vi "Drive.vi"(9 "JoystickDevRef 2":T1, 10 "JoystickDevRef":T1, 11 "RobotDriveDevRef":T3={"DevStatus"={"status"=FALSE, "code"=0, "source"=""}, "Motors[]"=[], "Square Inputs"=FALSE, "Max Output"=1.0}) -> (1 "JoystickDevRef 4":T1, 2 "JoystickDevRef 3":T1, 3 "RobotDriveDevRef 2":T3={"DevStatus"={"status"=FALSE, "code"=0, "source"=""}, "Motors[]"=[], "Square Inputs"=FALSE, "Max Output"=1.0})   [LabVIEW 2019]
uses:
  <vilib>/Rock Robotics/WPI/Joystick/WPI_JoystickDevRef.ctl
  <vilib>/Rock Robotics/WPI/Joystick/WPI_JoystickDeviceEnum.ctl
  <vilib>/Rock Robotics/WPI/RobotDrive/WPI_RobotDriveDevRef.ctl
  <vilib>/Rock Robotics/WPI/MotorControl/WPI_MotorControlDeviceRef.ctl
  <vilib>/Rock Robotics/WPI/MotorControl/WPI_MotorControlType.ctl
  <vilib>/Rock Robotics/SystemInterfaces/DIO/FPGA_DIOPWMChannel.ctl
  <vilib>/Rock Robotics/WPI/PWM/WPI_PWMDeadband.ctl
  <vilib>/Rock Robotics/SystemInterfaces/DIO/FPGA_DIOChannel.ctl
  Robot Global Data.vi
  <vilib>/Rock Robotics/WPI/Utilities/WPI_GetSetVariantRefNum.vi
  <vilib>/Rock Robotics/Network Tables/NT Read Number.vi
  <vilib>/Rock Robotics/WPI/RobotDrive/WPI_RobotDriveArcadeDrive_Standard(NoSaturation).vi
panel:
  in  "Double":dbl=0.5
  in  "Plus":dbl=0.2
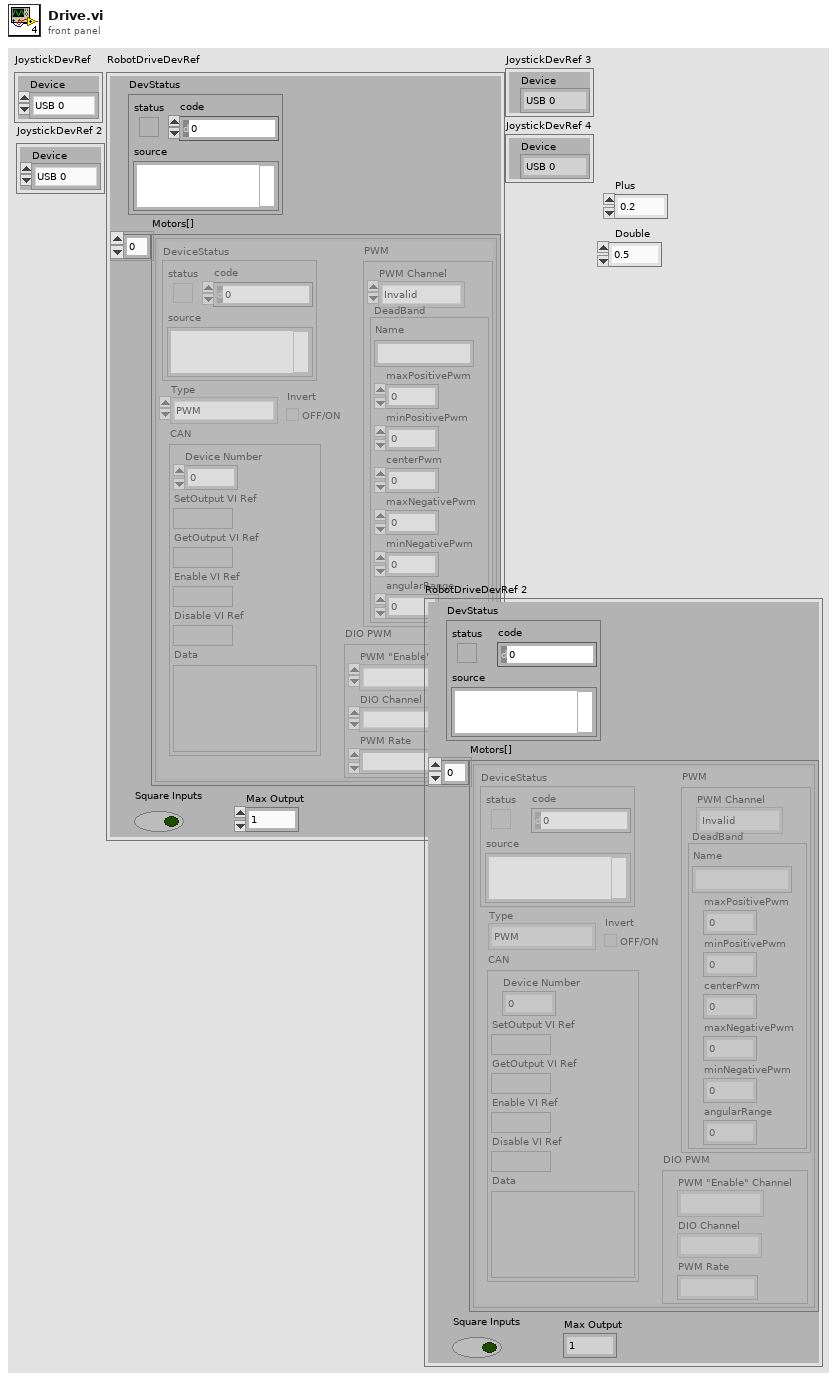
[diagram p1: front panel]
types:
  T1 = typedef "WPI_JoystickDevRef.ctl" = cluster{"Device":T2}
  T2 = typedef "WPI_JoystickDeviceEnum.ctl" = enum16{"USB 0", "USB 1", "USB 2", "USB 3", "USB 4", "USB 5"}
  T3 = typedef "WPI_RobotDriveDevRef.ctl" = cluster{"DevStatus":errorcluster, "Motors[]":T4[], "Square Inputs":bool, "Max Output":dbl}
  T4 = typedef "WPI_MotorControlDeviceRef.ctl" = cluster{"DeviceStatus":errorcluster, "Type":T5, "PWM":cluster{"PWM Channel":T6, "DeadBand":T7}, "CAN":cluster{"Device Number":u8, "SetOutput VI Ref":variant, "GetOutput VI Ref":variant, "Enable VI Ref":variant, "Disable VI Ref":variant, "Data":variant}, "Invert":bool, "DIO PWM":cluster{"PWM \"Enable\" Channel":T6, "DIOChannel":T8, "PWM Rate":dbl}}
  T5 = typedef "WPI_MotorControlType.ctl" = enum16{"PWM", "CAN", "DIO PWM"}
  T6 = typedef "FPGA_DIOPWMChannel.ctl" = enum8{"PWM 0", "PWM 1", "PWM 2", "PWM 3", "PWM 4", "PWM 5", "PWM 6", "PWM 7", "PWM 8", "PWM 9", "PWM MXP 0", "PWM MXP 1", "PWM MXP 2", "PWM MXP 3", "PWM MXP 4", "PWM MXP 5", "PWM MXP 6", "PWM MXP 7", "PWM MXP 8", "PWM MXP 9", "Invalid"}
  T7 = typedef "WPI_PWMDeadband.ctl" = cluster{"Name":string, "maxPositivePwm":i32, "minPositivePwm":i32, "centerPwm":i32, "maxNegativePwm":i32, "minNegativePwm":i32, "angularRange":u16}
  T8 = typedef "FPGA_DIOChannel.ctl" = enum8{"DIO 0", "DIO 1", "DIO 2", "DIO 3", "DIO 4", "DIO 5", "DIO 6", "DIO 7", "DIO 8", "DIO 9", "DIO MXP 0", "DIO MXP 1", "DIO MXP 2", "DIO MXP 3", "DIO MXP 4", "DIO MXP 5", "DIO MXP 6", "DIO MXP 7", "DIO MXP 8", "DIO MXP 9", "DIO MXP 10", "DIO MXP 11", "DIO MXP 12", "DIO MXP 13", "DIO MXP 14", "DIO MXP 15", "SPI Port CS1", "SPI Port CS2", "SPI Port CS3", "SPI Port MISO", "SPI Port MOSI", "Invalid"}
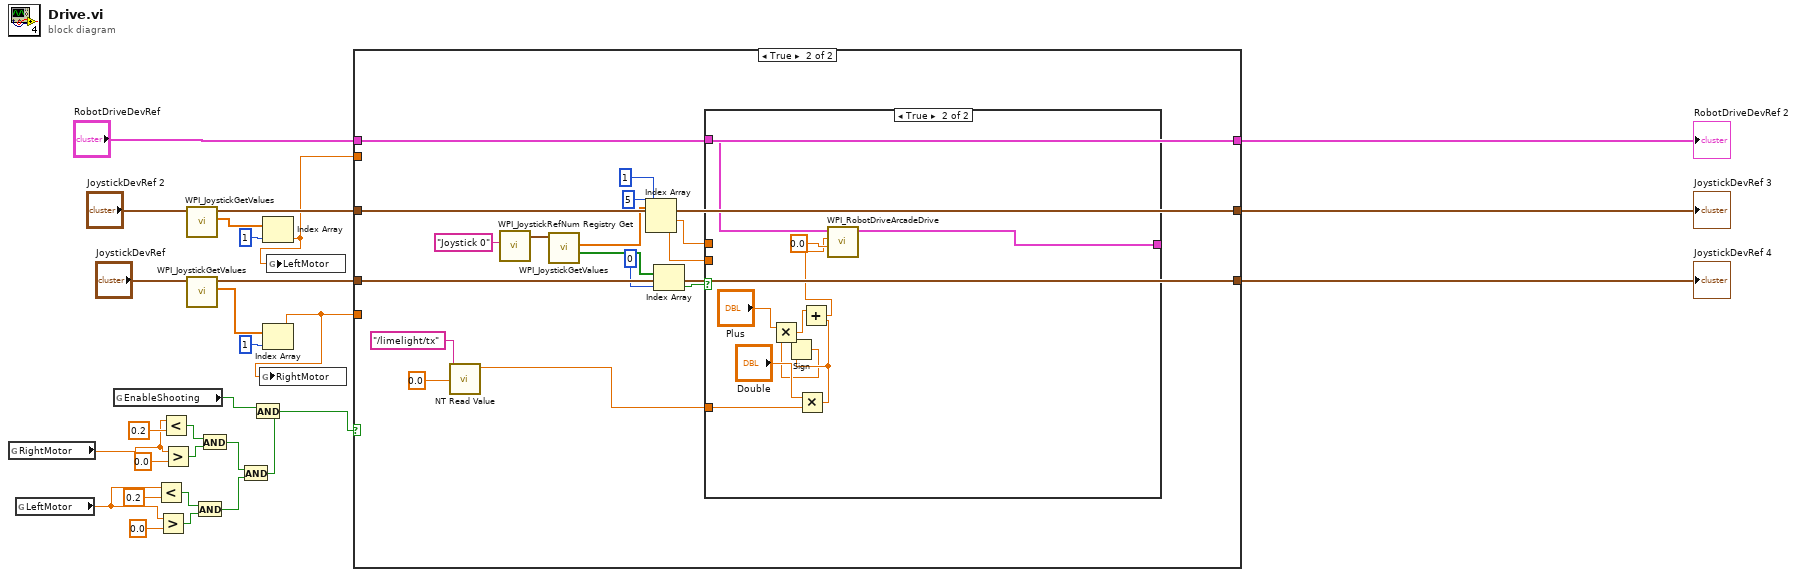
[diagram p0: block diagram]
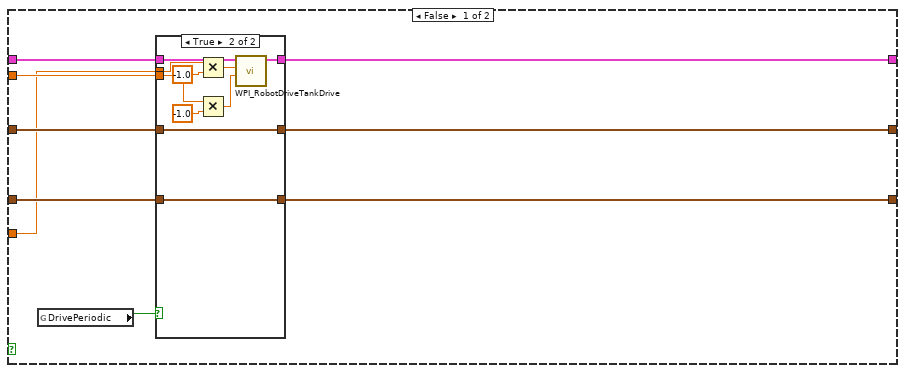
[diagram p2: hidden frame]
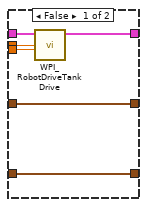
[diagram p3: hidden frame]
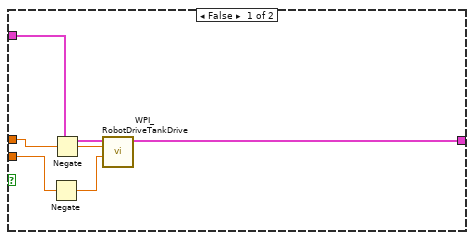
[diagram p4: hidden frame]
diagram:
  n1 = global read "Robot Global Data.vi" "RightMotor"() -> (w5:dbl)
  n2 = global read "Robot Global Data.vi" "LeftMotor"() -> (w11:dbl)
  n3 = global read "Robot Global Data.vi" "EnableShooting"() -> (w18:bool)
  n4 = Less?(x=w11, y=0.2) -> (x < y?=w12:bool)
  n5 = Greater?(x=w11, y=0.0) -> (0:w13:bool)
  n6 = Less?(x=w5, y=0.2) -> (x < y?=w7:bool)
  n7 = Greater?(x=w5, y=0.0) -> (0:w8:bool)
  n8 = call <vilib>:"WPI_JoystickGetValues.vi"("JoystickDevRef"="JoystickDevRef 2") -> ("Axes"=w28:dbl[], "JoystickDevRef"=w25:T1)  [unwired: 6 in, 3 out]
  n9 = call <vilib>:"WPI_JoystickGetValues.vi"("JoystickDevRef"="JoystickDevRef") -> ("Axes"=w29:dbl[], "JoystickDevRef"=w19:T1)  [unwired: 6 in, 3 out]
  n10 = And(x=w12, y=w13) -> (x .and. y?=w4:bool)
  n11 = And(x=w7, y=w8) -> (x .and. y?=w3:bool)
  n12 = And(x=w3, y=w4) -> (x .and. y?=w2:bool)
  n13 = And(x=w18, y=w2) -> (x .and. y?=w17:bool)
  n14 = Index Array(array=w28, index=1) -> (element=w16:dbl)
  n15 = Index Array(array=w29, index=1) -> (element=w15:dbl)
  n16 = global write "Robot Global Data.vi" "RightMotor"(w15) -> ()
  n17 = global write "Robot Global Data.vi" "LeftMotor"(w16) -> ()
  n18 = case shown="True" w17 {
    tunnel: w16 -> [w38 _]
    tunnel: w25 -> [w37 w69]
    tunnel: [w36 w55] -> w22
    tunnel: [w35 w69] -> w21
    tunnel: [w34 w70] -> w20
    tunnel: "RobotDriveDevRef" -> [w33 w55]
    tunnel: w19 -> [w31 w70]
    tunnel: w15 -> [w30 _]
    frame False {
      n19 = global read "Robot Global Data.vi" "DrivePeriodic"() -> (w32:bool)
      n20 = case shown="True" w32 {
        tunnel: w30 -> [w44 w52]
        tunnel: w38 -> [w43 w50]
        tunnel: [w42 w48] -> w36
        tunnel: w37 -> [w41 w47]
        tunnel: w31 -> [w40 w46]
        tunnel: [w40 w46] -> w34
        tunnel: [w41 w47] -> w35
        tunnel: w33 -> [w39 w45]
        frame False {
          n21 = call <vilib>:"WPI_RobotDriveTankDrive.vi"("Right axis value"=w43, "Left axis value"=w44, "RobotDriveDevRef"=w39) -> ("RobotDriveDevRef"=w42:T3)  [unwired: 6 in, 2 out]
        }
        frame True {
          n22 = Multiply(x=w52, y=-1.0) -> (x*y=w51:dbl)
          n23 = Multiply(x=w50, y=-1.0) -> (x*y=w49:dbl)
          n24 = call <vilib>:"WPI_RobotDriveTankDrive.vi"("Right axis value"=w49, "Left axis value"=w51, "RobotDriveDevRef"=w45) -> ("RobotDriveDevRef"=w48:T3)  [unwired: 6 in, 2 out]
        }
      }
    }
    frame True {
      n25 = call-poly <vilib>:"NT Read Value.vi"("Default Value"=0.0, "Name"="/limelight/tx") -> ("Numeric"=w56:dbl)  [unwired: 8 in, 1 out]
      n26 = call <vilib>:"WPI_JoystickRefNum Registry Get.vi"("refnum name"="Joystick 0") -> ("JoystickDevRef"=w67:T1)  [unwired: 9 in, 1 out]
      n27 = call <vilib>:"WPI_JoystickGetValues.vi"("JoystickDevRef"=w67) -> ("Buttons"=w66:bool[], "Axes"=w63:dbl[])  [unwired: 6 in, 3 out]
      n28 = Index Array(array=w63, index #1=1 ("index"), index #2=5 ("index")) -> (element #1=w60:dbl, element #2=w59:dbl)
      n29 = Index Array(array=w66, index=0) -> (element=w65:bool)
      n30 = case shown="True" w65 {
        tunnel: w55 -> [w76 w86]
        tunnel: w60 -> [w72 _]
        tunnel: w59 -> [w74 _]
        tunnel: [w75 w84] -> _
        tunnel: w56 -> [_ w81]
        frame False {
          n31 = Negate(x=w74) -> (-x=w73:dbl)
          n32 = Negate(x=w72) -> (-x=w71:dbl)
          n33 = call <vilib>:"WPI_RobotDriveTankDrive.vi"("Right axis value"=w73, "Left axis value"=w71, "RobotDriveDevRef"=w76) -> ("RobotDriveDevRef"=w75:T3)  [unwired: 6 in, 2 out]
        }
        frame True {
          n34 = Multiply(x="Double", y=w81) -> (x*y=w78:dbl)
          n35 = Sign(1:w78) -> (0:w77:dbl)
          n36 = Multiply(x="Plus", y=w77) -> (x*y=w79:dbl)
          n37 = Add(x=w79, y=w78) -> (x+y=w82:dbl)
          n38 = call-poly <vilib>:"WPI_RobotDriveArcadeDrive.vi"("Y axis value"=0.0, "X axis value"=w82, "RobotDriveDevRef"=w86) -> ("RobotDriveDevRef"=w84:T3)  [unwired: 6 in, 2 out]
        }
      }
    }
  }
  "RobotDriveDevRef 2" <- w22
  "JoystickDevRef 3" <- w21
  "JoystickDevRef 4" <- w20
